vi "Lockin.DAQ.GetPublicEvents.vi"(8 "error in (no error)":errorcluster, 11 "Lockin.DAQ":refnum<class "Lockin.DAQ.lvclass">) -> (0 "error out":errorcluster, 2 "LIADAQ Public Events":T1, 3 "Lockin.DAQ out":refnum<class "Lockin.DAQ.lvclass">)   [LabVIEW 2016, in "Lockin.DAQ.lvclass"]
doc: "---------------------------------------------------------------\nJKI State Machine Objects™\nhttp://jki.net/state-machine-objects/\nCopyright (C) 2005-2015, JKI <info@jki.net>\nALL RIGHTS RESERVEDJKI State Machine Objects (SMO) 1.0.0.4\nJKI - JKI\nCopyright (c) 2015, JKI"
uses:
  Lockin.DAQ.lvclass
  Typedefs/PublicEvents--Cluster.ctl
  Typedefs/PublicEvents--Lockin.DAQ.getAO.ctl
  Typedefs/PublicEvents--Lockin.DAQ.getAI.ctl
  Typedefs/PublicEvents--Lockin.DAQ.getREF.ctl
  Typedefs/PublicEvents--Lockin.DAQ.getResults.ctl
  Typedefs/Results--Cluster.ctl
  Typedefs/PublicEvents--Lockin.DAQ.getCalibration.ctl
  Typedefs/Cal Info - Cluster.ctl
  Typedefs/PublicEvents--Lockin.DAQ.getAOChannels.ctl
  Typedefs/AO-cluster.ctl
  Instrument.Lockinl.UI/Typedefs/AO Channel--Cluster.ctl
  Typedefs/Function-enum.ctl
  Typedefs/PublicEvents--Lockin.DAQ.getREFChannels.ctl
  Typedefs/REF-cluster.ctl
  Instrument.Lockinl.UI/Typedefs/REF Channel--Cluster.ctl
  Typedefs/PublicEvents--Lockin.DAQ.getDAQState.ctl
  Typedefs/State-enum.ctl
  Typedefs/PublicEvents--Lockin.DAQ.getSweepResults.ctl
  Typedefs/SweepResults--Cluster.ctl
  Typedefs/PublicEvents--Lockin.DAQ.getSweepWaveforms.ctl
  Typedefs/PublicEvents--Lockin.DAQ.getDAQconfig.ctl
  Instrument.Lockinl.UI/Typedefs/Device Configuration--Cluster.ctl
  Typedefs/446xAO-enum.ctl
  Typedefs/446xAI-enum.ctl
  Typedefs/AI.coupling-enum.ctl
  Lockin.DAQ.lvclass/Lockin.DAQ.ctl
  Instrument.Lockinl.UI/Instrument.Lockin.UI.lvclass
panel:
  # "For instructions on how to use the JKI State Machine Objects, examples and video tutorials, visit:\nhttp://jki.net/state-machine-objects/\n\nJKI State Machine Objects™\nhttp://jki.net/state-machine-objects/\nCopyright (C) 2005-2015, JKI <info@jki.net>\nALL RIGHTS RESERVED"
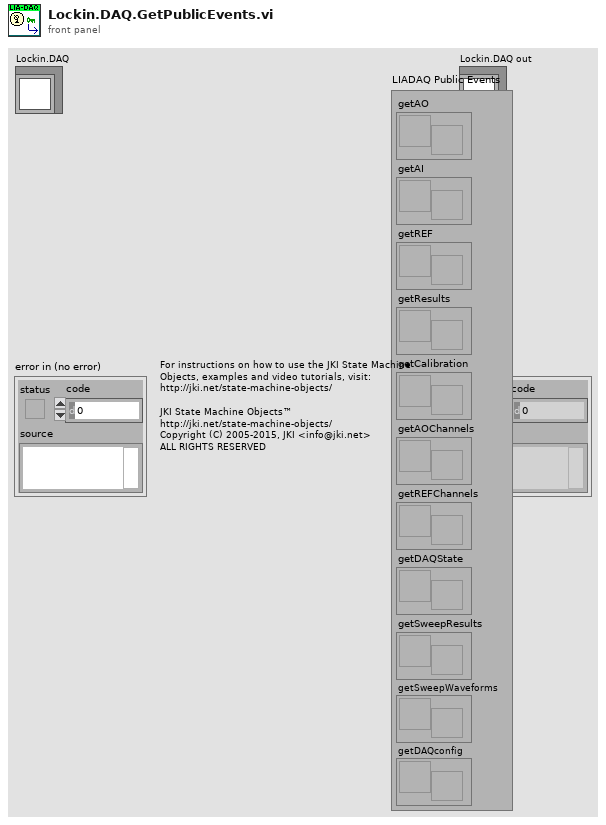
[diagram p1: front panel]
types:
  T1 = typedef "Lockin.DAQ.lvclass/PublicEvents--Cluster.ctl" = cluster{"getAO":refnum<user-event>, "getAI":refnum<user-event>, "getREF":refnum<user-event>, "getResults":refnum<user-event>, "getCalibration":refnum<user-event>, "getAOChannels":refnum<user-event>, "getREFChannels":refnum<user-event>, "getDAQState":refnum<user-event>, "getSweepResults":refnum<user-event>, "getSweepWaveforms":refnum<user-event>, "getDAQconfig":refnum<user-event>}
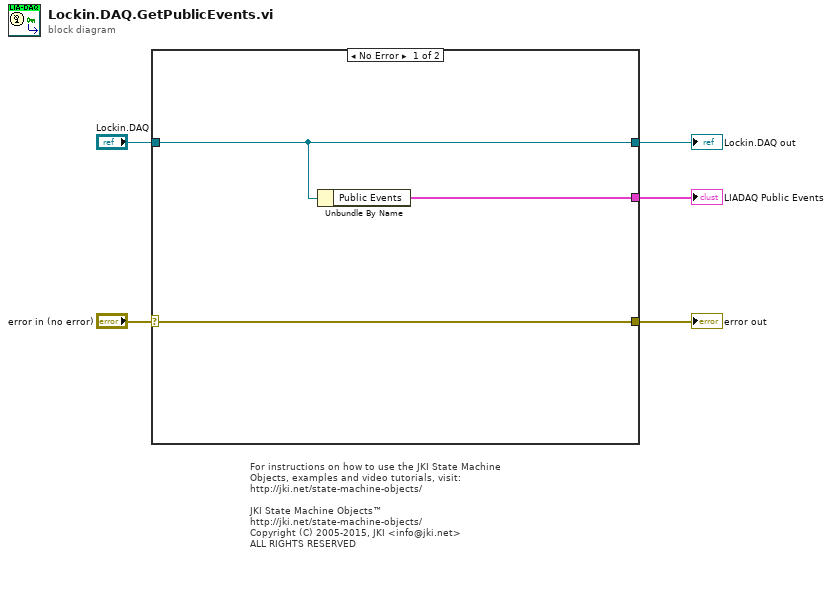
[diagram p0: block diagram]
diagram:
  # "For instructions on how to use the JKI State Machine Objects, examples and video tutorials, visit:\nhttp://jki.net/state-machine-objects/\n\nJKI State Machine Objects™\nhttp://jki.net/state-machine-objects/\nCopyright (C) 2005-2015, JKI <info@jki.net>\nALL RIGHTS RESERVED"
  n1 = case shown="No Error" "error in (no error)" {
    selector: "error in (no error)" -> [w7 w9]
    tunnel: "Lockin.DAQ" -> [w6 w10]
    tunnel: [w7 w9] -> w4
    tunnel: [w6 w10] -> w3
    tunnel: [w8 _] -> w1
    frame No Error {
      n2 = Unbundle By Name(w6) -> ("Public Events"=w8:T1)
    }
    frame Error {
    }
  }
  "error out" <- w4
  "Lockin.DAQ out" <- w3
  "LIADAQ Public Events" <- w1
